vi "2014_FireEveryNov11thAt111111.vi"(8 "error in (no error)":errorcluster) -> (0 "error out":errorcluster)   [LabVIEW 2013]
uses:
  source/Cron.Jenkins/Cron.Jenkins.lvclass/Cron.Jenkins.ctl
  source/Cron.Jenkins/Write Job Name.vi
  <vilib>/addons/_JKI Toolkits/Caraya/classes/Assert/Assert True.vi
  source/Cron/Create Cron Job.vi
  source/Cron/Compute Next Cron.vi
  source/Cron.Jenkins/Cron.Jenkins.lvclass
  <vilib>/addons/_JKI Toolkits/Caraya/classes/Test/Test.lvclass
  <vilib>/addons/_JKI Toolkits/Caraya/classes/Assert/Assert.lvclass
  source/openCron.lvlib
panel:
  out "Occurences":timestamp[](array[timestamp])
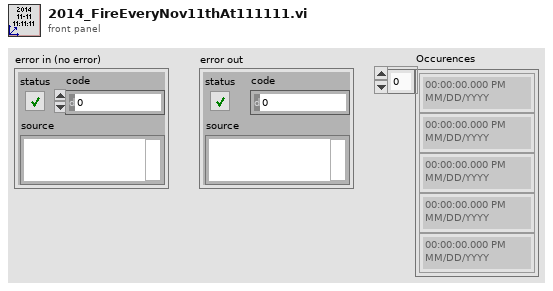
[diagram p1: front panel]
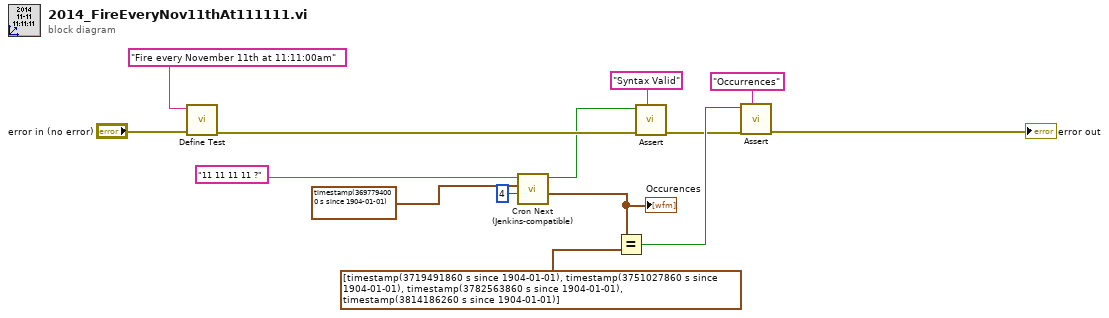
[diagram p0: block diagram]
diagram:
  n1 = call <vilib>:"Define Test.vi"("error in (no error)"="error in (no error)", "Label (VI Title)"="Fire every November 11th at 11:11:00am") -> ("error out"=w12:errorcluster)  [unwired: 9 in]
  n2 = call "Cron Next (Jenkins-compatible).vi"("Nb Occurences (min: 1)"=u16 4, "Reference timestamp (Now)"=timestamp(3697794000 s since 1904-01-01) ("y"), "Cron Expression"="11 11 11 11 ?" ("Expression")) -> ("Occurences"=w8:timestamp[], "syntax valid?"=w9:bool)  [unwired: 6 in, 1 out]
  "Occurences" <- w8
  n3 = Equal?(x=w8, y=timestamp[] [timestamp(3719491860 s since 1904-01-01), timestamp(3751027860 s since 1904-01-01), timestamp(3782563860 s since 1904-01-01), timestamp(3814186260 s since 1904-01-01)]) -> (x = y?=w11:bool)
  n4 = call-poly <vilib>:"Assert.vi"("Label"="Syntax Valid" ("Label (VI Title)"), "error in (no error)"=w12, "True?"=w9) -> ("error out"=w10:errorcluster)  [unwired: 8 in]
  n5 = call-poly <vilib>:"Assert.vi"("Label"="Occurrences" ("Label (VI Title)"), "error in (no error)"=w10, "True?"=w11) -> ("error out"=→"error out":errorcluster)  [unwired: 8 in]
